vi "LookupCommandPointer.vi"(11 "refnum name":string) -> (0 "error out":errorcluster, 3 "VI Refnum Out":refnum<vi>)   [LabVIEW 2015]
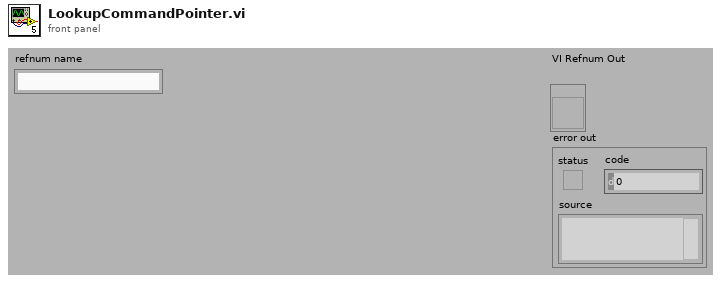
[diagram p1: front panel]
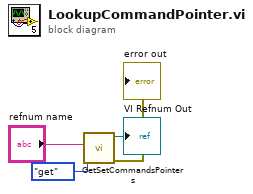
[diagram p0: block diagram]
diagram:
  n1 = call "GetSetCommandsPointers.vi"("menu"=enum16{"set", "get", "delete"}."get", "refnum name"="refnum name") -> ("error out"=→"error out":errorcluster, "VI Refnum Out"=→"VI Refnum Out":refnum<vi>)  [unwired: 2 in, 6 out]
